vi "SetCounter.vi"(8 "CtrEdge":u8, 9 "CtrMode":u8=1, 10 "CtrNum":u8, 11 "error in":errorcluster caption="错误输入") -> (3 "error out":errorcluster caption="错误输出")   [LabVIEW 2016]
uses:
  PLC-Lab/lib/gusb.dll
panel:
  # "CtrNum：计数器索引，255代表索引全部4个Counter"
  # "CtrMode：Counter模式，0-计数器，1-测周期，2-测正脉宽，3-测负脉宽"
  # "CtrEdge：计数器模式时，1-计上升沿，2-计下降沿"
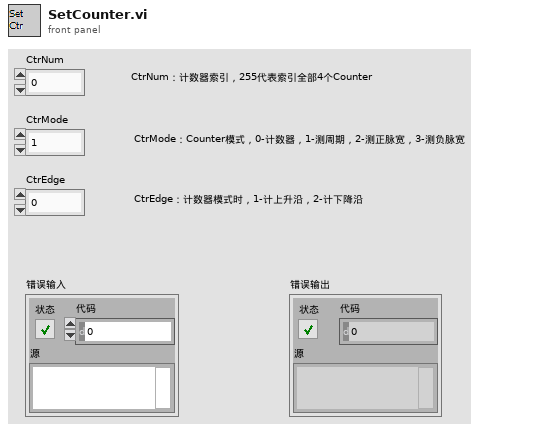
[diagram p1: front panel]
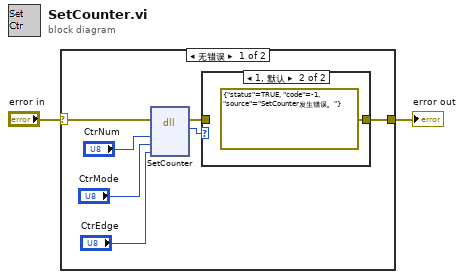
[diagram p0: block diagram]
diagram:
  n1 = case shown="无错误" "error in" {
    selector: "error in" -> [w9 w12]
    tunnel: [w7 w12] -> w1
    frame No Error {
      n2 = dll-call lib="E:/Camproject/2018/2018.1Labview/PLC-Lab/lib/gusb.dll" fn="SetCounter"(error in=w9, "CtrNum"="CtrNum", "CtrMode"="CtrMode", "CtrEdge"="CtrEdge") -> (error out=w6:errorcluster, "Status"=w8:i32)  [unwired: 5 in, 1 out]
      n3 = case shown="1, 默认" w8 {
        tunnel: w6 -> [w10 _]
        tunnel: [w10 errorcluster {"status"=TRUE, "code"=-1, "source"="SetCounter发生错误。"} ("错误常量")] -> w7
        frame 0 {
        }
        frame 1, Default {
        }
      }
    }
    frame Error {
    }
  }
  "error out" <- w1
